vi "Generate Reference File.vi"(0 "pBrightImage":u16[](array[numeric]), 1 "nWidth":u32, 2 "nHeight":u32, 5 "pDarkImage":u16[](array[numeric]), 9 "lpszSavePath":u8[](array[numeric]), 11 "error in":errorcluster, 12 "Acquisition Mode":T1) -> (4 "function return":i32, 15 "error out":errorcluster)   [LabVIEW 2022 SP3, in "BonTechDetector.lvlib"]
uses:
  BonTechDetector.lvlib
  BonTechWrapperLibrary.dll
  Controls/Acquisition Modes.ctl
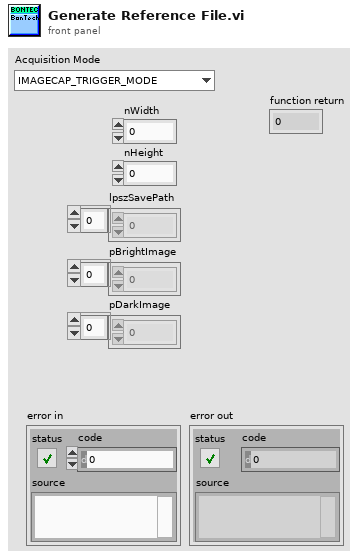
[diagram p1: front panel]
types:
  T1 = typedef "BonTechDetector.lvlib/Acquisition Modes.ctl" = enum32{"IMAGECAP_TRIGGER_MODE", "IMAGECAP_AED_MODE", "IMAGECAP_SOFTTRIGGER_MODE", "IMAGECAP_AVG_COUNT_MODE", "IMAGECAP_AVG_AED_MODE", "IMAGECAP_CONTINUOUS_MODE", "IMAGECAP_VIEWER_MODE", "IMAGECAP_CONTINUOUS_BINNING_MODE"}
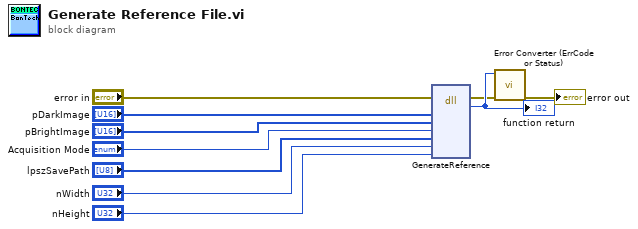
[diagram p0: block diagram]
diagram:
  n1 = dll-call lib="E:/SourceCodes/image-harvest/ImageHandler/BonTechDetector/BonTechWrapperLibrary.dll" fn="GenerateReference"(error in="error in", "pDarkImage"="pDarkImage", "pBrightImage"="pBrightImage", "nAcqMode"="Acquisition Mode", "lpszSavePath"="lpszSavePath", "nWidth"="nWidth", "nHeight"="nHeight") -> (error out=w5:errorcluster, "return type"=w6:i32)  [unwired: 8 in, 1 out]
  "function return" <- w6
  n2 = call "Error Converter (ErrCode or Status).vi"("error in (no error)"=w5, "error code"=w6) -> ("error out"=→"error out":errorcluster)  [unwired: 9 in]
